vi "injectJobClassInstance.vi"(8 "error in (no error)":errorcluster, 10 "Job":refnum<class "Job.lvclass">, 11 "VI in":refnum<vi>) -> (0 "error out":errorcluster, 3 "VI out":refnum<vi>)   [LabVIEW 2013, in "openCronJob.lvlib" / "Job.StaticVIRef.lvclass"]
uses:
  Job.StaticVIRef.lvclass
  Job/Job.lvclass
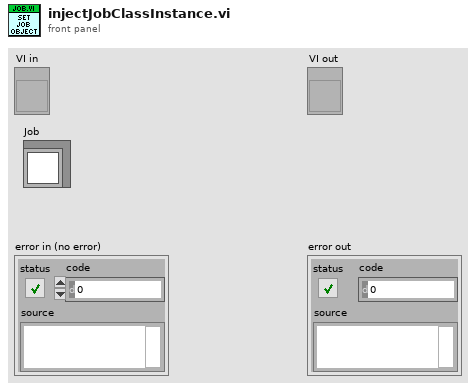
[diagram p1: front panel]
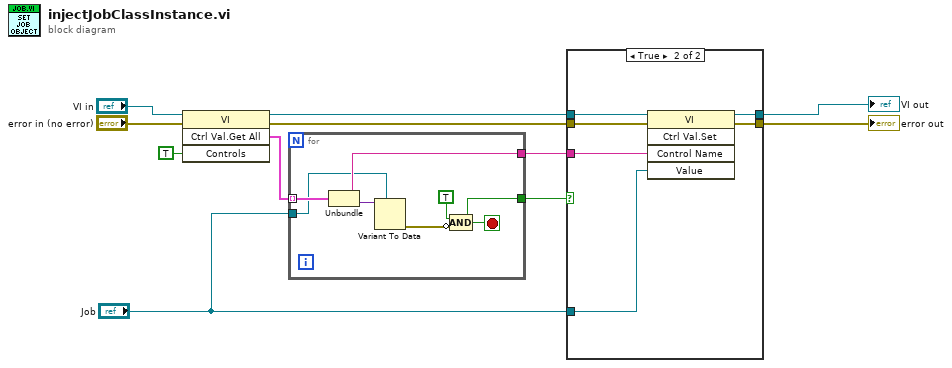
[diagram p0: block diagram]
diagram:
  n1 = invoke class="VI" method="Ctrl Val.Get All"(reference="VI in", error in="error in (no error)", "Controls"=TRUE) -> (reference out=w7:refnum<vi>, error out=w5:errorcluster, "Get All Control Values Variant"=w4:cluster{"Name":string, "Variant Data":variant}[])  [unwired: 1 in, 1 out]
  n2 = for {
    tunnel: w4 -> [w18] mode=indexing
    tunnel: "Job" -> [w13]
    tunnel: [w15] -> w3
    tunnel: [w14] -> w2
    stop <- w15 stop-if-true
    n3 = Unbundle(w18) -> ("Name"=w14:string, "Variant Data"=w17:variant)
    n4 = Variant To Data(type=w13, Variant=w17) -> (error out=w16:errorcluster)  [unwired: 1 in, 1 out]
    n5 = Compound Arithmetic op=AND(TRUE, invert w16) -> (w15:bool)
  }
  n6 = case shown="True" w3 {
    tunnel: [w19 w26] -> w11
    tunnel: [w20 w25] -> w10
    tunnel: w7 -> [w20 w24]
    tunnel: w5 -> [w19 w23]
    tunnel: "Job" -> [_ w22]
    tunnel: w2 -> [_ w21]
    frame False {
    }
    frame True {
      n7 = invoke class="VI" method="Ctrl Val.Set"(reference=w24, error in=w23, "Control Name"=w21, "Value"=w22) -> (reference out=w25:refnum<vi>, error out=w26:errorcluster)  [unwired: 1 in, 3 out]
    }
  }
  "error out" <- w11
  "VI out" <- w10
